vi "YeeToEye.vi"() -> ()   [LabVIEW 2022 SP3]
panel:
  in  "Case Constant\n(See Context Help)":bool=TRUE
  in  "Use Selected Files":bool
  in  "Listbox":i32[](listbox)
  in  "Choose Directory":path
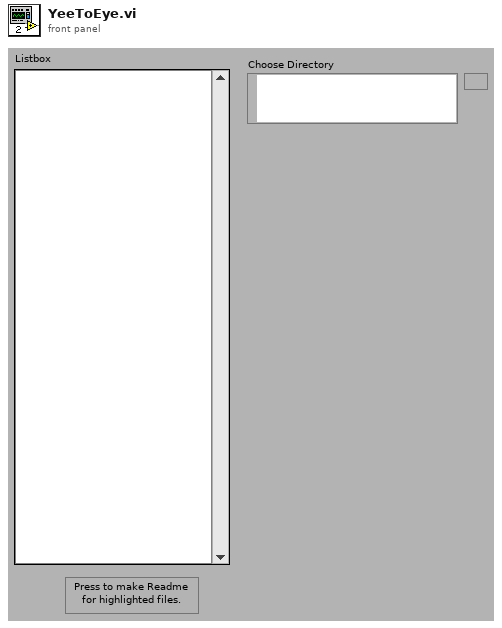
[diagram p1: front panel]
types:
  T1 = typedef "Header.ctl" = cluster{"header info":cluster{"Header":string, "Head length":i16}, "A/D info":cluster{"# rf points per line":u16, "# lines per scan":u16, "sample rate MHz":u16, "# A/D bits":i16, "# bytes per A/D":u16, "TGC Flag":u16, "A/D Type":string}, "Tranducer Info":cluster{"bandwidth":sgl, "center freq":sgl, "start freq":sgl, "ID":i32}, "Scan Info":cluster{"delay":sgl, "pivot distance":sgl, "sector scan angle":sgl, "operator":string, "Scan Mode":string, "location":string}, "Time/Date Info":cluster{"date":string, "time":string}, "RF Info":cluster{"RF file name":string, "RF file att":string, "RF cal file name":string, "RF cal file att":string}, "Patient Info":cluster{"ID":string, "extended ID":string, "age":u16, "sex":string, "previously\nscanned":string, "PSA":sgl, "LOS":u8, "Ethnicty 2":u8, "Race":u8}, "Tissue Type":cluster{"organ":i16, "disease type":i16, "disease location":i16, "IQ_pts":u16, "RcvBuffer":u8, "RcvFrame":u16, "IQBuff":u8, "IQFrame":u16, "IQPage":u8}, "Votage scaling":cluster{"Digitizer (dB)":sgl, "Gain (dB)":sgl, "Atten (dB)":sgl}, "Comment":string, "Misc Info":cluster{"avg num":u16, "c speed":i16, "Div By or SF zones":i16, "XMIT CHS":u8, "RCV CHS":u8, "Xmit angle":sgl}, "Therapy Parameters":cluster{"Theraputic Freq (MHz)":sgl, "Time on (s)":sgl, "Therapy amplitude (mV)":sgl, "Lines Before":u16, "Lines After":u16}, "Scan Settings":cluster{"Energy (uJ or V)":u8, "Damp (Ohm) or Fc":u8, "HP Filt (KHz)":u8, "LP Filt (MHz)":u8, "Gain (db)":u8, "prf (kHz)":sgl, "Distance between\nscan lines (um)":u16, "Distance between\nscan planes (um)":u16, "Scan line gap (um)":sgl, "Scan plane gap (um)":sgl}, "Compression Parameters":cluster{"F1 (MHz)":sgl, "F2 (MHz)":sgl, "% taper":sgl, "duration":sgl}, "Patient Info Xtra":cluster{"First Name":string, "Last Name":string, "Notes":string}, "ROI Box":u16[]}
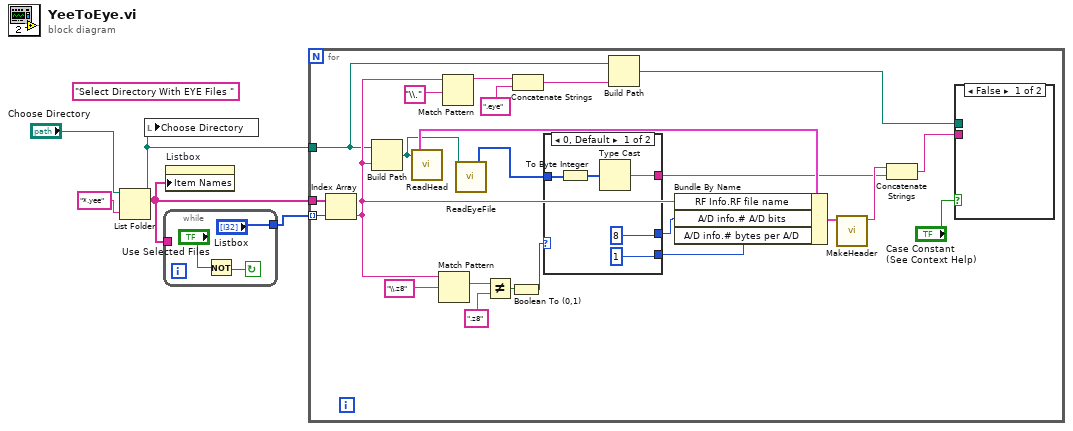
[diagram p0: block diagram]
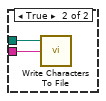
[diagram p2: hidden frame]
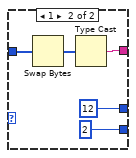
[diagram p3: hidden frame]
diagram:
  (unwired) "Select Directory With EYE Files " ("prompt")
  n1 = List Folder(path="Choose Directory", pattern="*.yee") -> (path out=w1:path, filenames=w4:string[])  [unwired: 1 in, 3 out]
  n2 = local write "Choose Directory"(w1) -> ()
  n3 = while {
    tunnel: ["Listbox"] -> w3
    tunnel: w4 -> [_]
    stop <- w8 continue-if-true
    n4 = Not(x="Use Selected Files") -> (.not. x?=w8:bool)
  }
  n5 = property on="Listbox" class="LstBox (strict)"("Item Names"=w4) -> ()  [unwired: 2 in, 2 out]
  n6 = for {
    tunnel: w4 -> [w32]
    tunnel: w3 -> [w31] mode=indexing
    tunnel: w1 -> [w14]
    n7 = Index Array(array=w32, index=w31) -> (element=w17:string)
    n8 = Build Path(base path=w14, name or relative path=w17) -> (appended path=w22:path)
    n9 = call "ReadHead.vi"("new file path"=w22) -> ("Header In"=w30:T1)  [unwired: 18 out]
    n10 = Match Pattern(string=w17, regular expression="\\.z8") -> (match substring=w29:string)  [unwired: 4 out]
    n11 = Match Pattern(string=w17, regular expression="\\.") -> (before substring=w16:string)  [unwired: 4 out]
    n12 = call "ReadEyeFile.vi"("new file path"=w22) -> ("1-D data"=w21:i16[])  [unwired: 1 in, 17 out]
    n13 = Not Equal?(x=w29, y=".z8") -> (x != y?=w27:bool)
    n14 = Boolean To (0,1)(Boolean=w27) -> (0, 1=w26:i16)
    n15 = Concatenate Strings(w16, ".eye") -> (w13:string)
    n16 = case shown="0, Default" w26 {
      tunnel: [8 12] -> w25
      tunnel: [1 2] -> w24
      tunnel: w21 -> [w36 w41]
      tunnel: [w35 w40] -> w19
      frame 0, Default {
        n17 = To Byte Integer(number=w36) -> (8bit integer=w37:i8[])
        n18 = Type Cast(x=w37) -> (*(type *) &x=w35:string)  [unwired: 1 out]
      }
      frame 1 {
        n19 = Swap Bytes(anything=w41) -> (byte swapped=w42:i16[])
        n20 = Type Cast(x=w42) -> (*(type *) &x=w40:string)  [unwired: 1 out]
      }
    }
    n21 = Build Path(base path=w14, name or relative path=w13) -> (appended path=w11:path)
    n22 = Bundle By Name(cluster=w30, "RF Info.RF file name"=w17, "A/D info.# A/D bits"=w25, "A/D info.# bytes per A/D"=w24) -> (w23:T1)
    n23 = call "MakeHeader.vi"("Header In"=w23) -> ("Header String"=w20:string)  [unwired: 6 out]
    n24 = Concatenate Strings(w20, w19) -> (w10:string)
    n25 = case shown="False" "Case Constant\n(See Context Help)" {
      tunnel: w11 -> [_ w34]
      tunnel: w10 -> [_ w33]
      frame False {
      }
      frame True {
        n26 = call <vilib>:"Write Characters To File.vi"("character string"=w33, "file path (dialog if empty)"=w34) -> ()  [unwired: 1 in, 3 out]
      }
    }
  }
